vi "Sort cantilever info metadata.vi"(0 "reference in":refnum<class "metadata.lvclass">, 5 "error in (no error)":errorcluster) -> (14 "reference out":refnum<class "metadata.lvclass">, 16 "Cantilever info":T1, 19 "error out":errorcluster)   [LabVIEW 2019, in "metadata.lvclass"]
uses:
  metadata.lvclass
  Cantilever info parameters.ctl
panel:
  out "Array":string[](array[string])
  out "Array 2":i32[](array[numeric])
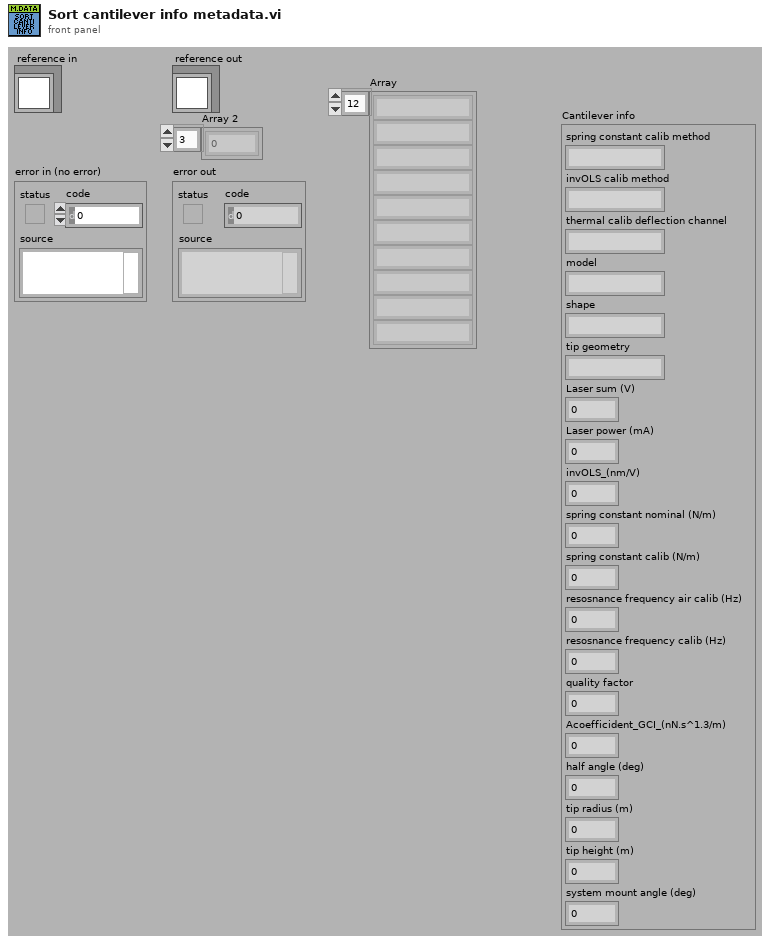
[diagram p1: front panel]
types:
  T1 = typedef "metadata.lvclass/Cantilever info parameters.ctl" = cluster{"spring constant calib method":string, "invOLS calib method":string, "thermal calib deflection channel":string, "model":string, "shape":string, "tip geometry":string, "Laser sum (V)":dbl, "Laser power (mA)":dbl, "invOLS_(nm/V)":dbl, "spring constant nominal (N/m)":dbl, "spring constant calib (N/m)":dbl, "resosnance frequency air calib (Hz)":dbl, "resosnance frequency calib (Hz)":dbl, "quality factor":dbl, "Acoefficident_GCI_(nN.s^1.3/m)":dbl, "half angle (deg)":dbl, "tip radius (m)":dbl, "tip height (m)":dbl, "system mount angle (deg)":dbl}
  T2 = typedef "metadata.lvclass/ObjectAttributesRef.ctl" = refnum<data-value>
  T3 = typedef "metadata.lvclass/ObjectAttributes.ctl" = cluster{"MyAttribute":dbl, "System Control":T4, "file info":T5, "Sample info":T6, "Cantilever info":T1, "XYZ piezos":T7, "Mapping":T8, "Fcurve segment":T9[], "Fast fpga segment":T11, "Chirp":T12, "precision (6)":i16, "width (-)":i16, "Metadata":T13, "config filepath":path, "Section names []":string[], "Property names []":string[], "nb elements":u16}
  T4 = typedef "metadata.lvclass/System control parameters.ctl" = cluster{"FPGA SW version":string, "TDMS file version":string, "Instrument":string, "Instrument model":string, "Instrument scanner":string, "Instrument clockrate (Mhz)":string, "Instrument tick time (us)":string}
  T5 = typedef "metadata.lvclass/File info parameters.ctl" = cluster{"Time Stamp":timestamp, "Filename":string, "Filepath":path, "User":string, "Experiment_name":string, "Curve_id":string, "number_segments":u8, "number_consecutive_scans":u32}
  T6 = typedef "metadata.lvclass/Sample info parameters.ctl" = cluster{"Sample name":string, "Sample species":string}
  T7 = typedef "metadata.lvclass/XYZ piezos parameters.ctl" = cluster{"X stage piezo sensitivity (nm/V)":dbl, "X stage piezo gain":dbl, "X velocity (V/tick)":dbl, "X closed loop":bool, "Y stage piezo sensitivity (nm/V)":dbl, "Y stage piezo gain":dbl, "Y velocity (V/tick)":dbl, "Y closed loop":bool, "Z stage piezo sensitivity (nm/V)":dbl, "Z stage piezo gain":dbl, "Z closed loop":bool, "X position (V)":dbl, "Y position (V)":dbl}
  T8 = typedef "metadata.lvclass/Mapping parameters.ctl" = cluster{"Mapping":bool, "index":u16, "position row":u16, "position column":u16, "next position row":i16, "next position column":i16, "X initial position (V)":dbl, "Y initial position (V)":dbl, "X step size (V)":dbl, "Y step size (V)":dbl}
  T9 = typedef "metadata.lvclass/Fcurve segment.ctl" = cluster{"type":T10, "fast_fpga_trigger":bool, "nb":u8, "duration (ticks)":i64, "nb points":i32, "sampling rate (S/s)":u32, "Zpiezo control out":string, "initial deflection (V)":dbl, "relative setpoint":bool, "setpoint on":bool, "setpoint (V)":dbl, "setpoint trigger channel":string, "velocity (V/tick)":dbl, "Z position setpoint trigger (V)":dbl, "Z retract length (V)":dbl, "dec factor":u32}
  T10 = typedef "metadata.lvclass/Segment type--combobox.ctl" = string
  T11 = typedef "metadata.lvclass/fast fpga segment parameters.ctl" = cluster{"Fast start time trigger":timestamp, "nb_points":u32, "sampling_rate_(S/s)":u32, "duration_(ticks)":u32}
  T12 = typedef "metadata.lvclass/Chirp added parameters.ctl" = cluster{"f start (Hz)":dbl, "f end (Hz)":dbl, "Sweep type":string}
  T13 = typedef "metadata.lvclass/Metadata output --cluster.ctl" = cluster{"Property Names":string[], "Property Values":variant[]}
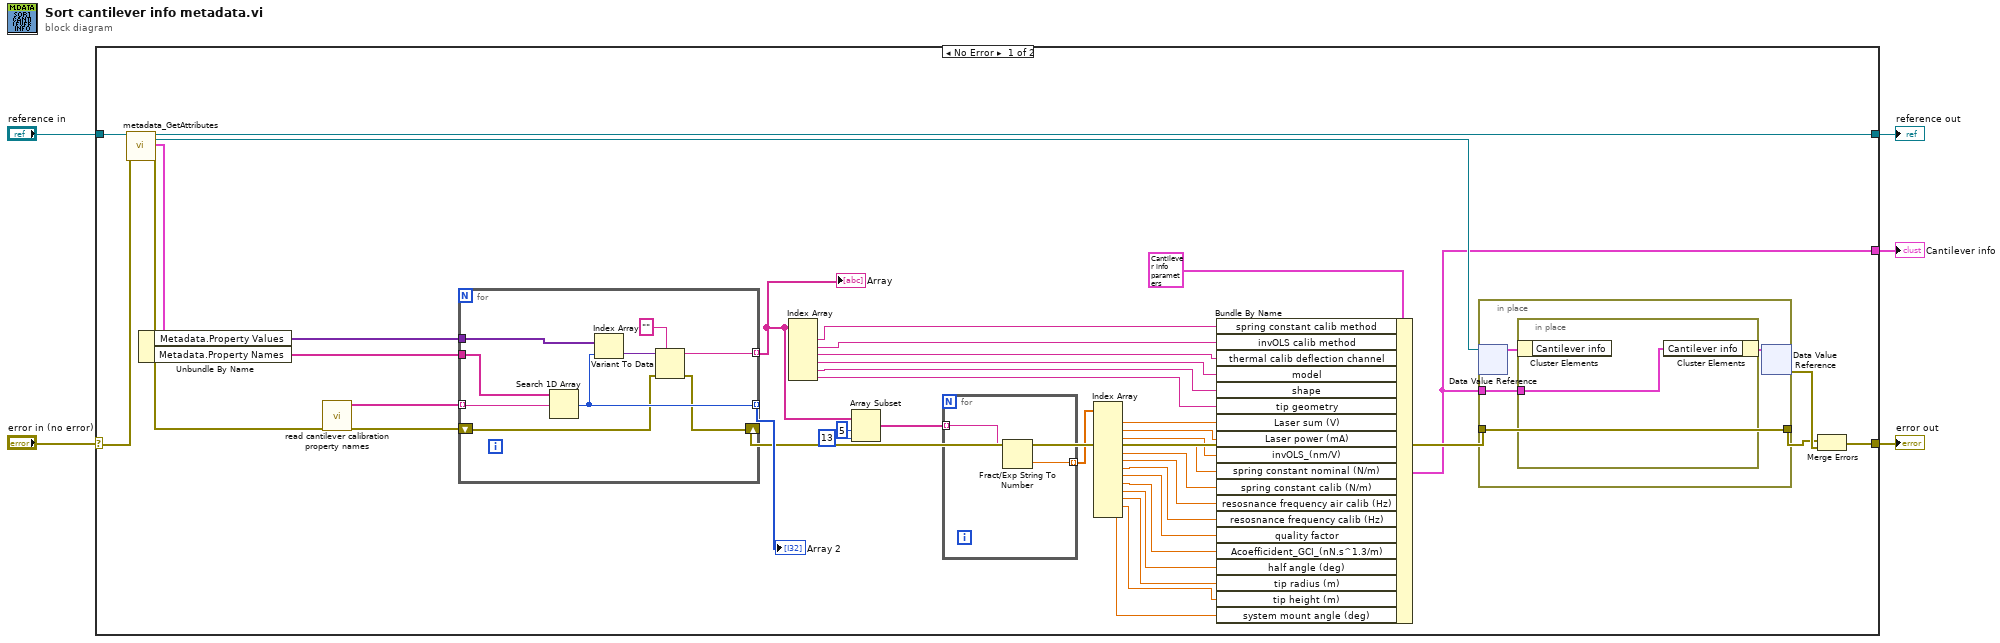
[diagram p0: block diagram]
diagram:
  n1 = case shown="No Error" "error in (no error)" {
    selector: "error in (no error)" -> [w42 w64]
    tunnel: [w46 w64] -> w4
    tunnel: [w41 w63] -> w2
    tunnel: "reference in" -> [w43 w63]
    tunnel: [w34 _] -> w1
    frame No Error {
      n2 = call "metadata_GetAttributes.vi"("reference in"=w43, "error in (no error)"=w42) -> ("reference out"=w41:refnum<class "metadata.lvclass">, "attributes ref"=w40:T2, "attributes"=w39:T3, "error out"=w8:errorcluster)  [unwired: 14 in]
      n3 = Unbundle By Name(w39) -> ("Metadata.Property Values"=w35:variant[], "Metadata.Property Names"=w38:string[])
      n4 = call "read cantilever calibration property names.vi"("error in (no error)"=w8) -> ("Cantilever calib"=w6:string[], "error out"=w7:errorcluster)  [unwired: 17 in]
      n5 = for {
        tunnel: w6 -> [w57] mode=indexing
        tunnel: [w54] -> w37 mode=indexing
        shift-right: [w50] -> w36
        shift-left: w7 -> [w51]
        tunnel: w38 -> [w56]
        tunnel: w35 -> [w55]
        tunnel: [w52] -> w26 mode=indexing
        n6 = Search 1D Array(1D array=w56, element=w57) -> (index of element=w54:i32)  [unwired: 1 in]
        n7 = Index Array(array=w55, index=w54) -> (element=w53:variant)
        n8 = Variant To Data(error in=w51, type="", Variant=w53) -> (data=w52:string, error out=w50:errorcluster)
      }
      "Array 2" <- w37
      "Array" <- w26
      n9 = Index Array(array=w26) -> (element #1=w32:string, element #2=w31:string, element #3=w30:string, element #4=w29:string, element #5=w28:string, element #6=w27:string)  [unwired: 6 in]
      n10 = Array Subset(array=w26, index=5, length=13) -> (w23:string[])
      n11 = for {
        tunnel: w23 -> [w48] mode=indexing
        tunnel: [w47] -> w22 mode=indexing
        n12 = Fract/Exp String To Number(string=w48) -> (number=w47:dbl)  [unwired: 3 in, 1 out]
      }
      n13 = Index Array(array=w22) -> (element #1=w21:dbl, element #2=w20:dbl, element #3=w19:dbl, element #4=w18:dbl, element #5=w17:dbl, element #6=w16:dbl, element #7=w15:dbl, element #8=w14:dbl, element #9=w13:dbl, element #10=w12:dbl, element #11=w11:dbl, element #12=w10:dbl, element #13=w9:dbl)  [unwired: 13 in]
      n14 = Bundle By Name(cluster=T1 {"spring constant calib method"="", "invOLS calib method"="", "thermal calib deflection channel"="", "model"="", "shape"="", "tip geometry"="", "Laser sum (V)"=0.0, "Laser power (mA)"=0.0, "invOLS_(nm/V)"=0.0, "spring constant nominal (N/m)"=0.0, "spring constant calib (N/m)"=0.0, "resosnance frequency air calib (Hz)"=0.0, "resosnance frequency calib (Hz)"=0.0, "quality factor"=0.0, "Acoefficident_GCI_(nN.s^1.3/m)"=0.0, "half angle (deg)"=0.0, "tip radius (m)"=0.0, "tip height (m)"=0.0, "system mount angle (deg)"=0.0} ("Cantilever info"), "spring constant calib method"=w32, "invOLS calib method"=w31, "thermal calib deflection channel"=w30, "model"=w29, "shape"=w28, "tip geometry"=w27, "Laser sum (V)"=w21, "Laser power (mA)"=w20, "invOLS_(nm/V)"=w19, "spring constant nominal (N/m)"=w18, "spring constant calib (N/m)"=w17, "resosnance frequency air calib (Hz)"=w16, "resosnance frequency calib (Hz)"=w15, "quality factor"=w14, "Acoefficident_GCI_(nN.s^1.3/m)"=w13, "half angle (deg)"=w12, "tip radius (m)"=w11, "tip height (m)"=w10, "system mount angle (deg)"=w9) -> (w34:T1)
      n15 = in-place {
        in-place-border: w36 -> [w59]
        in-place-border: [w59] -> w44
        in-place-border: w34 -> [w58]
        n16 = in-place-dvr #1(w40) -> (w60:T3)  [unwired: 1 out]
        n17 = in-place {
          in-place-border: w58 -> [w62]
          n18 = in-place-cluster #2(w60) -> ()  [unwired: 1 out]
          n19 = in-place-cluster #2("Cantilever info"=w62) -> (w61:T3)
        }
        n20 = in-place-dvr #1(w61) -> (w45:errorcluster)  [unwired: 1 out]
      }
      n21 = Merge Errors(w44, w45) -> (w46:errorcluster)
    }
    frame Error {
    }
  }
  "error out" <- w4
  "reference out" <- w2
  "Cantilever info" <- w1
